vi "Message Get.vi"(1 "Timeout ms (-1)":i32=-1, 2 "Module":string) -> (0 "data out":string)   [LabVIEW 2009]
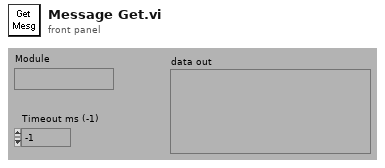
[diagram p1: front panel]
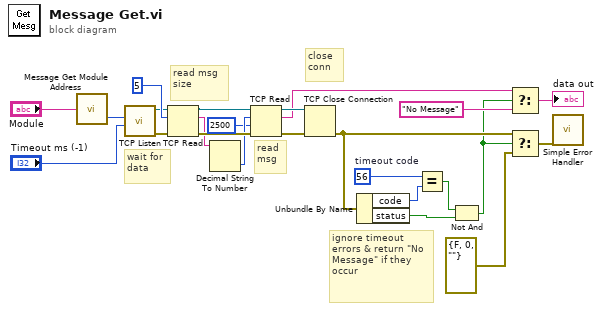
[diagram p0: block diagram]
diagram:
  w12 = 56  # timeout code
  # "close conn"
  # "ignore timeout errors & return \"No Message\" if they occur"
  # "wait for data"
  # "read msg"
  # "read msg size"
  n1 = call "Message Get Module Address.vi"("Module"="Module") -> ("Port"=w24:u16)  [unwired: 1 out]
  n2 = call <vilib>:"TCP Listen.vi"("timeout ms (wait forever: -1)"="Timeout ms (-1)", "port"=w24) -> ("error out"=w17:errorcluster, "connection ID"=w16:refnum<k5>)  [unwired: 6 in, 2 out]
  n3 = TCP Read(connection ID=w16, bytes to read=5 ("size of message length"), error in (no error)=w17) -> (connection ID out=w21:refnum<k5>, data out=w19:string, error out=w22:errorcluster)  [unwired: 2 in]
  n4 = Decimal String To Number(string=w19) -> (number=w20:i32)  [unwired: 2 in, 1 out]
  n5 = TCP Read(connection ID=w21, bytes to read=w20, error in (no error)=w22, 9:2500 ("timeout ms (25000)")) -> (connection ID out=w13:refnum<k5>, data out=w5:string, error out=w14:errorcluster)  [unwired: 1 in]
  n6 = TCP Close Connection(connection ID=w13, error in (no error)=w14) -> (error out=w7:errorcluster)  [unwired: 1 in, 1 out]
  n7 = Unbundle By Name(w7) -> ("code"=w11:i32, "status"=w9:bool)
  n8 = Equal?(x=w12, y=w11) -> (x = y?=w10:bool)
  n9 = Not And(1:w9, 2:w10) -> (0:w3:bool)
  n10 = Select(t=w5, s=w3, f="No Message") -> (s? t:f=→"data out":string)
  n11 = Select(t=w7, s=w3, f=errorcluster {"status"=FALSE, "code"=0, "source"=""} ("error out")) -> (s? t:f=w6:errorcluster)
  n12 = call <vilib>:"Simple Error Handler.vi"("error in (no error)"=w6) -> ()  [unwired: 4 in, 5 out]
